vi "Edit-action.vi"(8 "error in (no error)":errorcluster, 9 "Position in":i32, 11 "Sequence in":refnum<class "Action-sequence.lvclass">) -> (0 "error out":errorcluster, 1 "Position":i32, 3 "Sequence out":refnum<class "Action-sequence.lvclass">)   [LabVIEW 2013, in "PowderDeposition.lvlib" / "Action-sequence.lvclass"]
uses:
  Action-sequence.lvclass
  Action/Action.lvclass
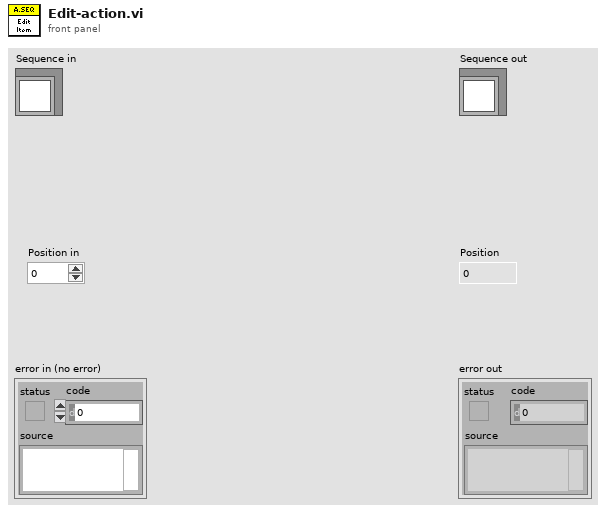
[diagram p1: front panel]
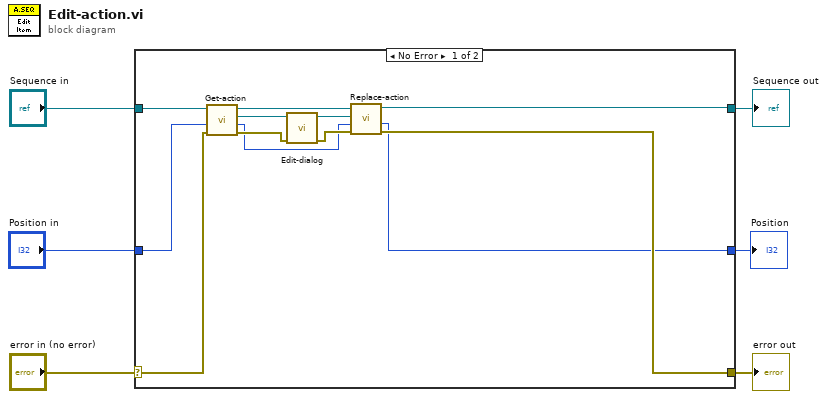
[diagram p0: block diagram]
diagram:
  n1 = case shown="No Error" "error in (no error)" {
    selector: "error in (no error)" -> [w16 w21]
    tunnel: [w9 w21] -> w5
    tunnel: [w10 w20] -> w3
    tunnel: "Sequence in" -> [w18 w20]
    tunnel: "Position in" -> [w17 w19]
    tunnel: [w7 w19] -> w1
    frame No Error {
      n2 = call "Get-action.vi"("error in (no error)"=w16, "Position in"=w17, "Sequence in"=w18) -> ("error out"=w14:errorcluster, "Position"=w8:i32, "Action"=w15:refnum<class "Action.lvclass">, "Sequence out"=w13:refnum<class "Action-sequence.lvclass">)  [unwired: 5 in]
      n3 = call-dynamic "Edit-dialog.vi"("error in (no error)"=w14, "Action in"=w15) -> ("error out"=w12:errorcluster, "Action out"=w11:refnum<class "Action.lvclass">)  [unwired: 8 in]
      n4 = call "Replace-action.vi"("error in (no error)"=w12, "Position in"=w8, "Action"=w11, "Sequence in"=w13) -> ("error out"=w9:errorcluster, "Position"=w7:i32, "Sequence out"=w10:refnum<class "Action-sequence.lvclass">)  [unwired: 4 in, 1 out]
    }
    frame Error {
    }
  }
  "error out" <- w5
  "Sequence out" <- w3
  "Position" <- w1
